vi "hse-application__SystemIdentifier.vi"(8 "error in (no error)":errorcluster) -> (0 "error out":errorcluster, 2 "System Identifier":string)   [LabVIEW 2020, in "hse-application.lvclass"]
doc: "____\nHAMPEL SOFTWARE ENGINEERING v3.8.0 (2023-12-18 14:41)"
uses:
  hse-application.lvclass
  kernel32.dll
  ole32.dll
  <resource>/objmgr/nisysapi.rc
  <vilib>/nisyscfg/nisyscfg.lvlib
  <vilib>/nisyscfg/Close (System).vi
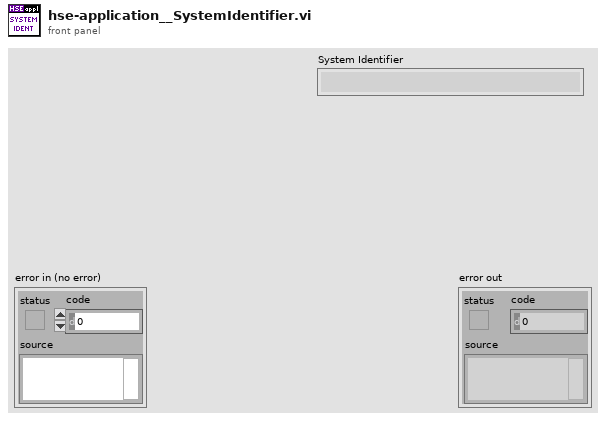
[diagram p1: front panel]
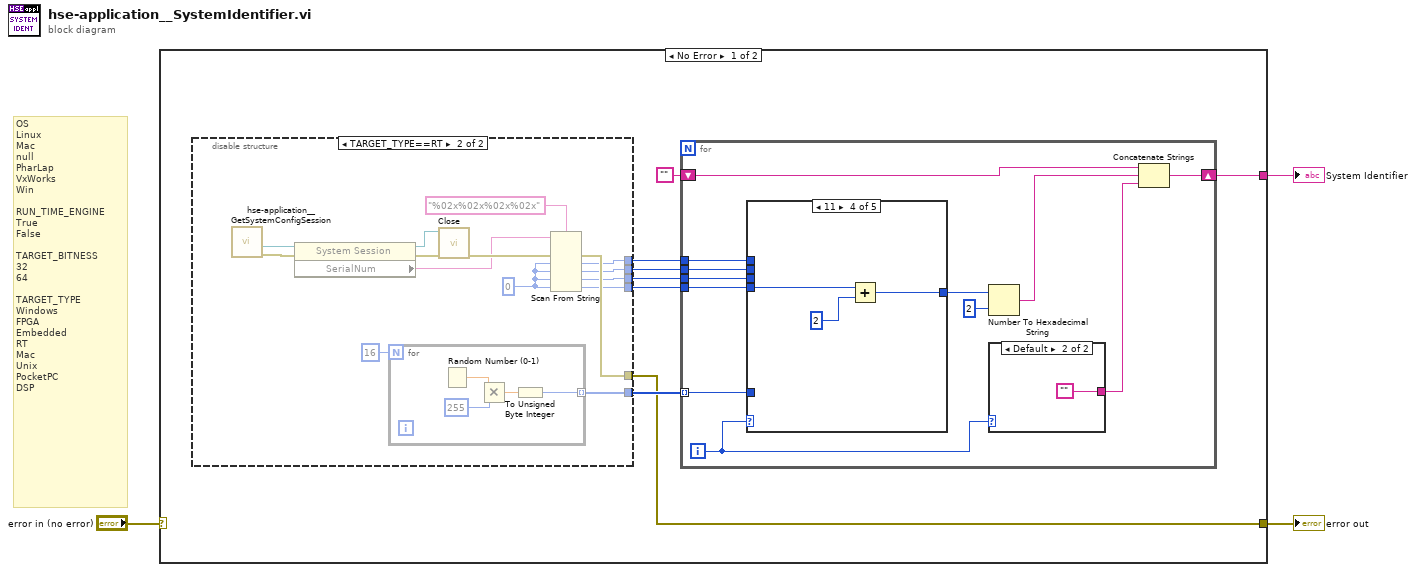
[diagram p0: block diagram]
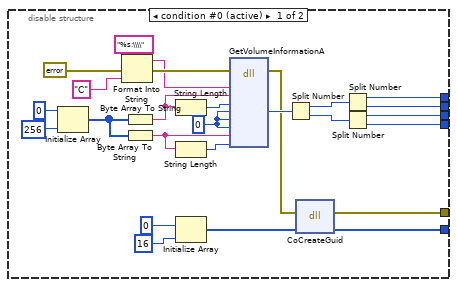
[diagram p2: hidden frame]
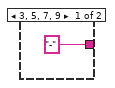
[diagram p3: hidden frame]
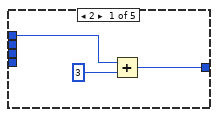
[diagram p4: hidden frame]
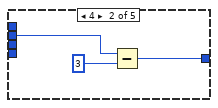
[diagram p5: hidden frame]
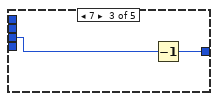
[diagram p6: hidden frame]
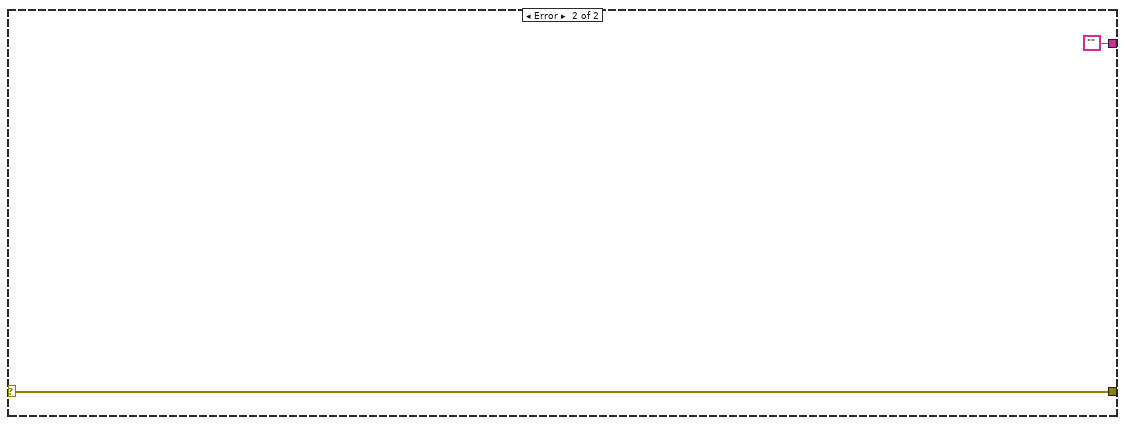
[diagram p8: hidden frame]
diagram:
  # "OS \nLinux\nMac\nnull\nPharLap\nVxWorks\nWin\n \nRUN_TIME_ENGINE \nTrue\nFalse \n\nTARGET_BITNESS \n32\n64 \n\nTARGET_TYPE \nWindows\nFPGA\nEmbedded\nRT\nMac\nUnix\nPocketPC\nDSP"
  n1 = case shown="No Error" "error in (no error)" {
    selector: "error in (no error)" -> [_ w84]
    tunnel: [w4 w84] -> w2
    tunnel: [w5 "" ("Empty String Constant")] -> w1
    frame No Error {
      n2 = disable-structure "Conditional Disable Structure" shown="TARGET_TYPE==RT" {
        disable-tunnel: [w24 w47] -> w11
        disable-tunnel: [w20 w40] -> w9
        disable-tunnel: [w19 w41] -> w8
        disable-tunnel: [w18 w42] -> w7
        disable-tunnel: [w17 w43] -> w6
        disable-tunnel: [w13 w45] -> w4
        frame condition #0 (active) {
          w30 = 0
          n3 = Initialize Array(u8 0 ("U8"), 256) -> (w35:u8[])
          n4 = Format Into String(format string="%s:\\\\", error in=errorcluster {"status"=FALSE, "code"=0, "source"=""}, "C" ("VOLUME (single character)")) -> (resulting string=w12:string, error out=w15:errorcluster)  [unwired: 1 in]
          n5 = Byte Array To String(unsigned byte array=w35) -> (string=w34:string)
          n6 = Byte Array To String(unsigned byte array=w35) -> (string=w32:string)
          n7 = String Length(string=w34) -> (length=w33:i32)
          n8 = String Length(string=w32) -> (length=w31:i32)
          n9 = Initialize Array(u8 0 ("element"), 16 ("dimension size")) -> (w25:u8[])
          n10 = dll-call lib="kernel32.dll" fn="GetVolumeInformationA"(error in=w15, "lpRootPathName"=w12, "lpVolumeNameBuffer"=w34, "nVolumeNameSize"=w33, "lpVolumeSerialNumber"=w30, "lpMaximumComponentLength"=w30, "lpFileSystemFlags"=w30, "lpFileSystemNameBuffer"=w32, "nFileSystemNameSize"=w31) -> (error out=w14:errorcluster, "lpVolumeSerialNumber"=w23:i32)  [unwired: 4 in, 7 out]
          n11 = Split Number(x=w23) -> (hi(x)=w22:u16, lo(x)=w21:u16)
          n12 = dll-call lib="ole32.dll" fn="CoCreateGuid"(error in=w14, "GUID"=w25) -> (error out=w13:errorcluster, "GUID"=w24:u8[])  [unwired: 3 in, 1 out]
          n13 = Split Number(x=w22) -> (hi(x)=w20:u8, lo(x)=w19:u8)
          n14 = Split Number(x=w21) -> (hi(x)=w18:u8, lo(x)=w17:u8)
        }
        frame condition #1 {
          w50 = u8 0 ("default value 1")
          n15 = call "hse-application__GetSystemConfigSession.vi"() -> ("error out"=w39:errorcluster, "Refnum out"=w38:refnum<k21>)  [unwired: 10 in]
          n16 = property on="Property Node" class="System Session"(reference=w38, error in=w39) -> (reference out=w52:refnum<k21>, error out=w51:errorcluster, "SerialNum"=w44:string)
          n17 = for {
            N: 16 -> [_]
            tunnel: [w53] -> w47 mode=indexing
            n18 = Random Number (0-1)() -> (number: 0 to 1=w56:dbl)
            n19 = Multiply(x=w56, y=u8 255 ("default value 1")) -> (x*y=w54:dbl)
            n20 = To Unsigned Byte Integer(number=w54) -> (unsigned 8bit integer=w53:u8)
          }
          n21 = call-poly <vilib>:"Close.vi"("error in (no error)"=w51, "Session in"=w52) -> ("error out"=w46:errorcluster)  [unwired: 9 in]
          n22 = Scan From String(format string="%02x%02x%02x%02x", input string=w44, error in=w46, default 1=w50, default 2=w50, default 3=w50, default 4=w50) -> (error out=w45:errorcluster, output 1=w40:u8, output 2=w41:u8, output 3=w42:u8, output 4=w43:u8)  [unwired: 1 in, 2 out]
        }
      }
      n23 = for {
        tunnel: w11 -> [w66] mode=indexing
        shift-right: [w61] -> w5
        shift-left: "" ("Empty String Constant") -> [w58]
        tunnel: w9 -> [w65]
        tunnel: w8 -> [w64]
        tunnel: w7 -> [w63]
        tunnel: w6 -> [w62]
        i -> [w59]
        n24 = case shown="11" w59 {
          tunnel: [w71 w75 w77 w80 w82] -> w67
          tunnel: w66 -> [_ _ _ _ w82]
          tunnel: w65 -> [w73 _ _ _ _]
          tunnel: w64 -> [_ w74 _ _ _]
          tunnel: w63 -> [_ _ w78 _ _]
          tunnel: w62 -> [_ _ _ w79 _]
          frame 2 {
            n25 = Add(x=w73, y=u8 3) -> (x+y=w71:u8)
          }
          frame 4 {
            n26 = Subtract(x=w74, y=u8 3) -> (x-y=w75:u8)
          }
          frame 7 {
            n27 = Decrement(x=w78) -> (x-1=w77:u8)
          }
          frame 11 {
            n28 = Add(x=w79, y=u8 2) -> (x+y=w80:u8)
          }
          frame Default {
          }
        }
        n29 = Number To Hexadecimal String(1:i16 2 ("width (-)"), 2:w67) -> (0:w57:string)
        n30 = case shown="Default" w59 {
          tunnel: ["-" "" ("Empty String Constant")] -> w60
          frame 3, 5, 7, 9 {
          }
          frame Default {
          }
        }
        n31 = Concatenate Strings(w58, w57, w60) -> (w61:string)
      }
    }
    frame Error {
    }
  }
  "error out" <- w2
  "System Identifier" <- w1
